vi "write data cell with column offset.vi"(5 "Column relative?":bool, 6 "Data Input":dbl, 7 "data column":i32=6, 8 "error in (no error)":errorcluster, 9 "row offset":i32, 10 "start of last occupied row":cluster{"row":i32, "column":i32}, 11 "NI_report in":refnum<class "NI_report.lvclass">) -> (0 "error out":errorcluster, 3 "NI_report out":refnum<class "NI_report.lvclass">)   [LabVIEW 2016]
uses:
  <vilib>/Utility/NIReport.llb/NI_report.lvclass
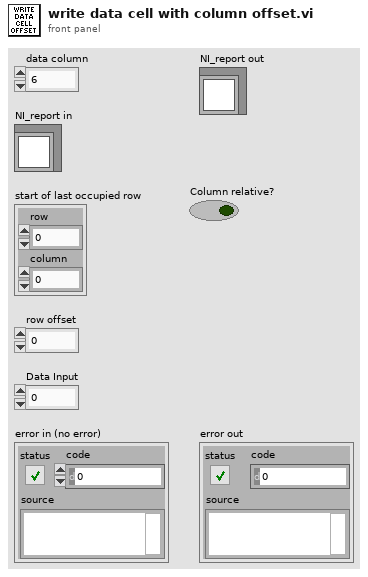
[diagram p1: front panel]
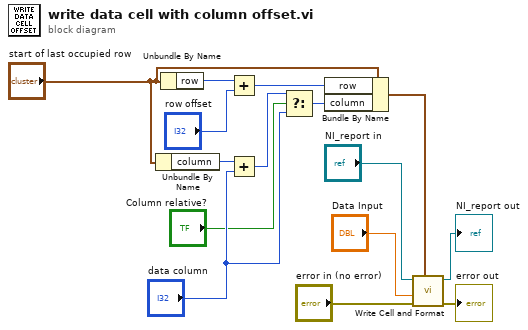
[diagram p0: block diagram]
diagram:
  n1 = Unbundle By Name("start of last occupied row") -> ("column"=w5:i32)
  n2 = Unbundle By Name("start of last occupied row") -> ("row"=w6:i32)
  n3 = Add(x=w6, y="row offset") -> (x+y=w11:i32)
  n4 = Add(x=w5, y="data column") -> (x+y=w3:i32)
  n5 = Select(t=w3, s="Column relative?", f="data column") -> (s? t:f=w4:i32)
  n6 = Bundle By Name(cluster="start of last occupied row", "row"=w11, "column"=w4) -> (w12:cluster{"row":i32, "column":i32})
  n7 = call "Write Cell and Format.vi"("output cluster"=w12, "error in (no error)"="error in (no error)", "Data In"="Data Input", "NI_report in"="NI_report in") -> ("error out"=→"error out":errorcluster, "NI_report out"=→"NI_report out":refnum<class "NI_report.lvclass">)  [unwired: 6 in]
